vi "ListVIs Reserved In Context.vi"() -> ()   [LabVIEW 2013]
panel:
  out "Not reserved anymore":string[](array[string])
  out "Reserved in this context":string[](array[string])
  out "Reserved in other context":string[](array[string])
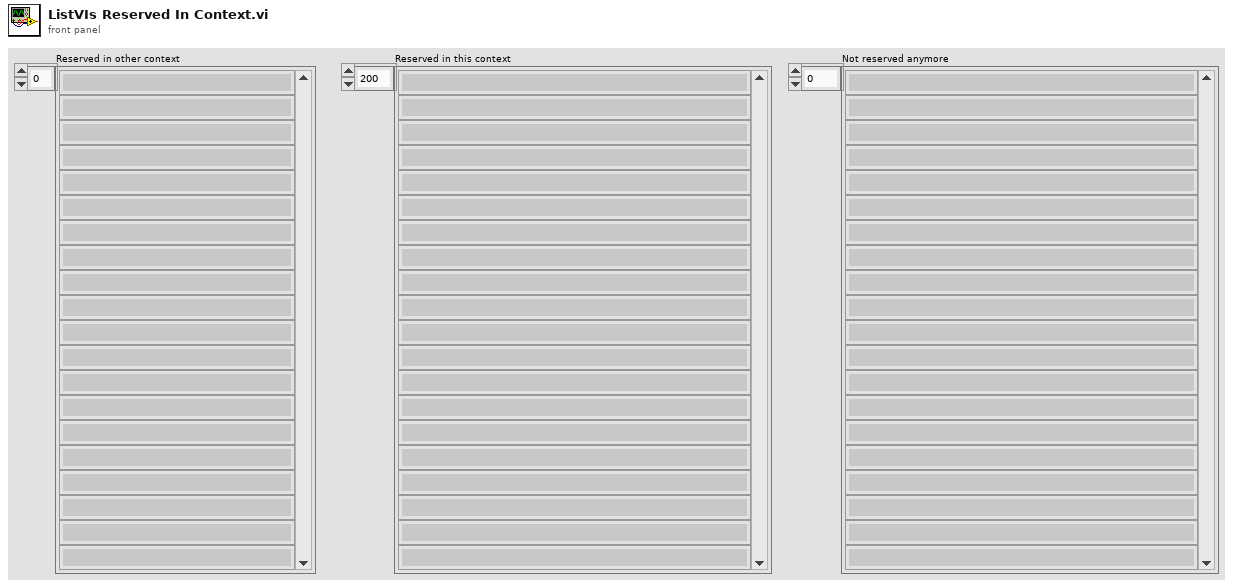
[diagram p1: front panel]
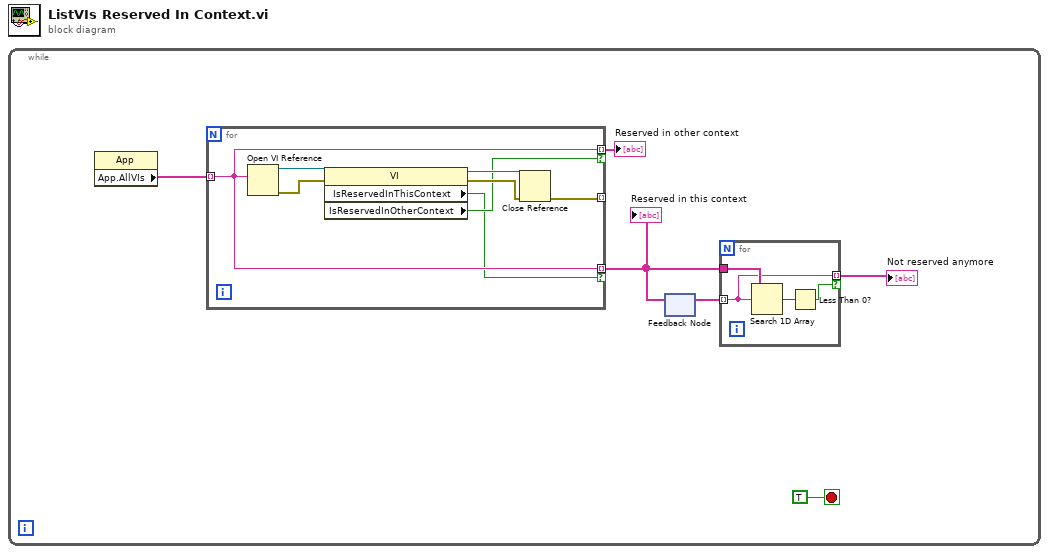
[diagram p0: block diagram]
diagram:
  n1 = while {
    stop <- TRUE stop-if-true
    n2 = property class="App"() -> ("App.AllVIs"=w6:string[])  [unwired: 2 in, 2 out]
    n3 = for {
      tunnel: w6 -> [w13] mode=indexing
      tunnel: [w13] -> w5 mode=indexing if=w12
      tunnel: [w16] -> _ mode=indexing
      tunnel: [w13] -> w1 mode=indexing if=w11
      n4 = Open VI Reference(vi path=w13) -> (vi reference=w18:refnum<vi>, error out=w15:errorcluster)  [unwired: 5 in]
      n5 = property class="VI"(reference=w18, error in=w15) -> (reference out=w17:refnum<vi>, error out=w14:errorcluster, "IsReservedInThisContext"=w11:bool, "IsReservedInOtherContext"=w12:bool)
      n6 = Close Reference(reference=w17, error in (no error)=w14) -> (error out=w16:errorcluster)
    }
    "Reserved in other context" <- w5
    "Reserved in this context" <- w1
    n7 = feedback-in #1(w1) -> ()
    n8 = feedback #1() -> (w3:string[])  [unwired: 1 in]
    n9 = for {
      tunnel: w3 -> [w7] mode=indexing
      tunnel: w1 -> [w8]
      tunnel: [w7] -> w2 mode=indexing if=w10
      n10 = Search 1D Array(1D array=w8, element=w7) -> (index of element=w9:i32)  [unwired: 1 in]
      n11 = Less Than 0?(x=w9) -> (x < 0?=w10:bool)
    }
    "Not reserved anymore" <- w2
  }
